vi "CloseSV.vi"(8 "error in (no error)":errorcluster, 11 "Shared variable refnum":refnum<k21>) -> (0 "error out":errorcluster)   [LabVIEW 2016, in "Shared Variable Interface.lvlib" / "DBL.lvlib"]
uses:
  DBL.lvlib
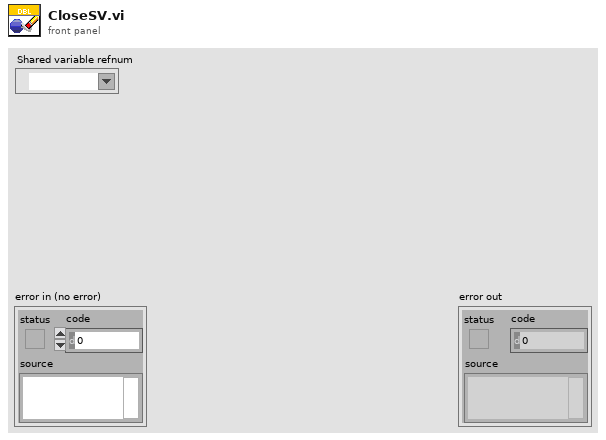
[diagram p1: front panel]
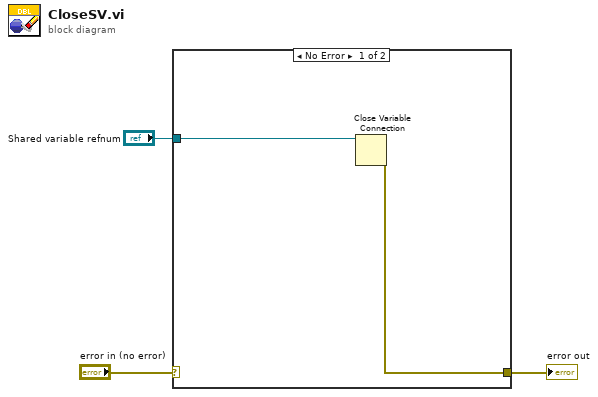
[diagram p0: block diagram]
diagram:
  n1 = case shown="No Error" "error in (no error)" {
    selector: "error in (no error)" -> [_ w6]
    tunnel: [w5 w6] -> w2
    tunnel: "Shared variable refnum" -> [w4 _]
    frame No Error {
      n2 = Close Variable Connection(11:w4) -> (0:w5:errorcluster)  [unwired: 1 in]
    }
    frame Error {
    }
  }
  "error out" <- w2
